vi "Time.vi"(8 "error in (no error)":errorcluster, 10 "Control In":T1, 11 "CAD Dispense in":refnum<class "CAD Dispense.lvclass">) -> (0 "error out":errorcluster, 1 "Timing Data":i32[](array[numeric]), 2 "Control Out":T1, 3 "CAD Dispense out":refnum<class "CAD Dispense.lvclass">)   [LabVIEW 2020, in "CAD Dispense.lvclass"]
uses:
  CAD Dispense.lvclass
  Controller/Motion/Motion.lvclass
  Controller/Controllers.ctl
  Controller/Controller.lvclass
  Controller/I-O/I-O.lvclass
  Controller/Dispenser/Dispenser.lvclass
  C:/Program Files (x86)/Aerotech/A3200/LabVIEW/2010/Bin/Aerotech.A3200.dll
  Program Files (x86)/Aerotech/A3200/LabVIEW/2010/Bin/Aerotech.A3200.dll
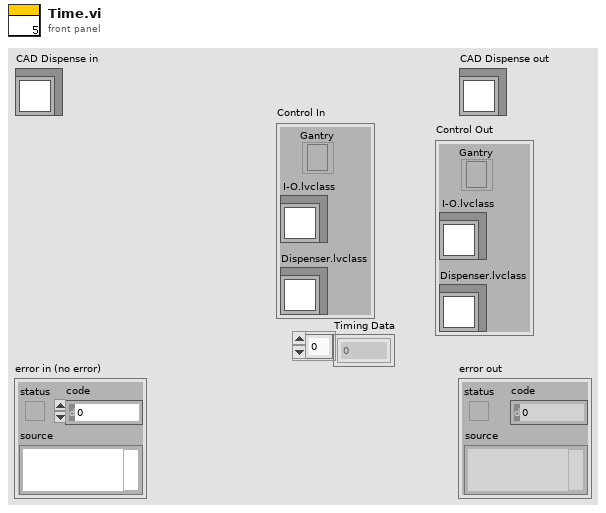
[diagram p1: front panel]
types:
  T1 = typedef "Controller.lvclass/Controllers.ctl" = cluster{"I-O.lvclass":refnum<class "I-O.lvclass">, "Dispenser.lvclass":refnum<class "Dispenser.lvclass">, "Gantry":refnum<k24>}
  T2 = cluster{"Motion":dbl[][], "Center":dbl[], "CW/CCW":dbl, "Dispense Type":enum16{"N-gon", "Square", "Arc", "Dot", "Line", "Circle"}}[]
  T3 = enum16{"N-gon", "Square", "Arc", "Dot", "Line", "Circle"}
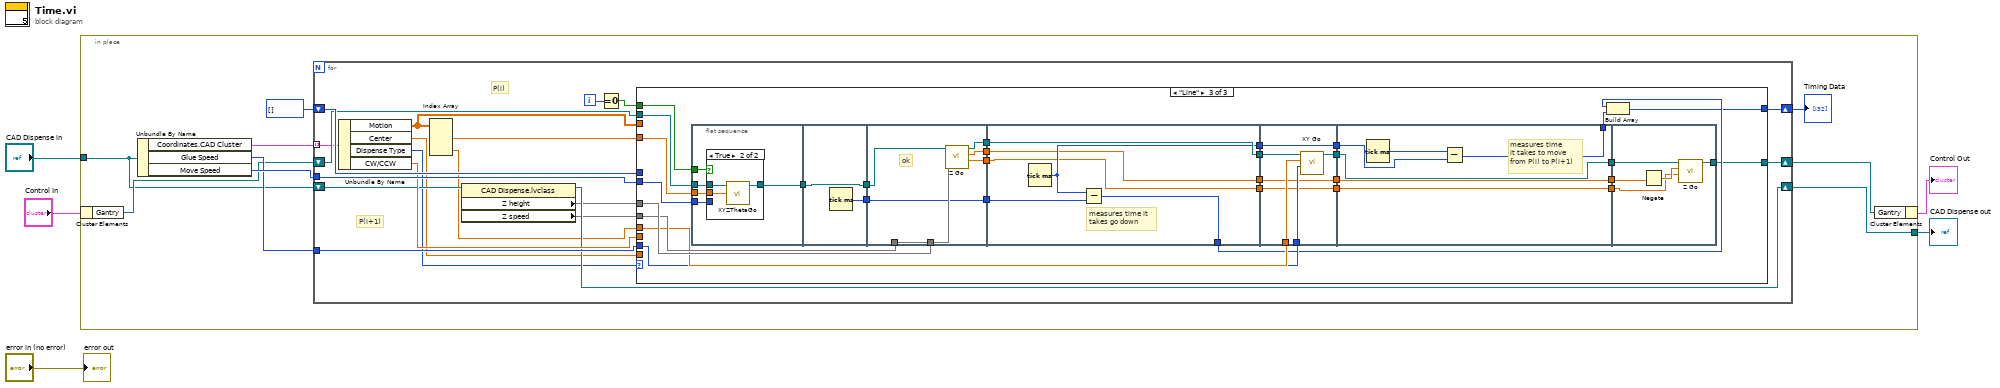
[diagram p0: block diagram]
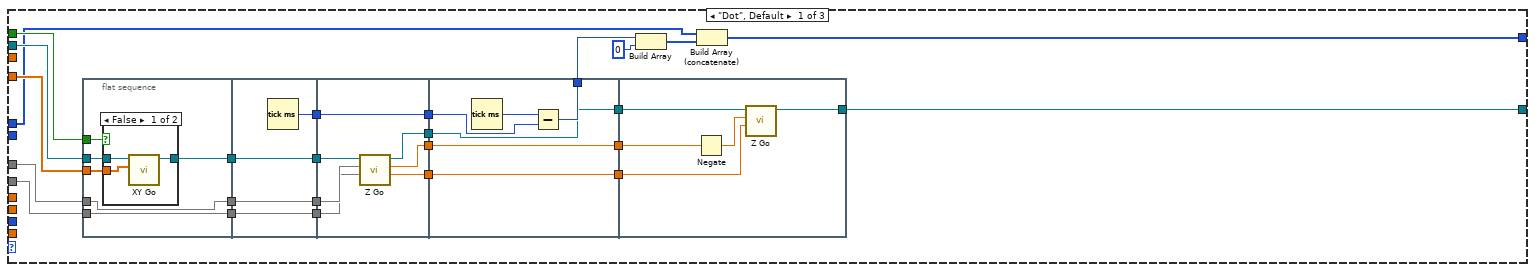
[diagram p2: hidden frame]
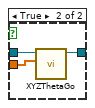
[diagram p3: hidden frame]
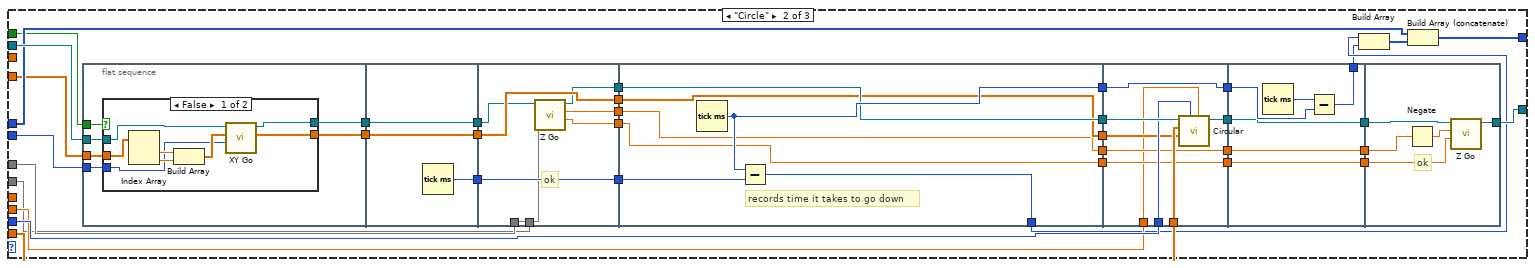
[diagram p4: hidden frame]
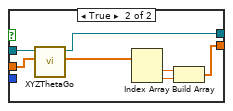
[diagram p5: hidden frame]
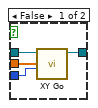
[diagram p6: hidden frame]
diagram:
  n1 = in-place {
    in-place-border: "CAD Dispense in" -> [w10]
    in-place-border: [w9] -> w1
    n2 = in-place-cluster #1("Control In") -> ("Gantry"=w11:refnum<k24>)
    n3 = Unbundle By Name "Unbundle By Name"(w10) -> ("Coordinates.CAD Cluster"=w6:T2, "Glue Speed"=w13:i32, "Move Speed"=w14:i32)
    n4 = for {
      tunnel: w14 -> [w33]
      shift-right: [w17] -> w7
      shift-left: w11 -> [w30]
      tunnel: w13 -> [w32]
      shift-right: [w22] -> w8
      shift-left: i32[] [] -> [w31]
      shift-right: [w27] -> w9
      shift-left: w10 -> [w28]
      tunnel: w6 -> [w21] mode=indexing
      i -> [w26]
      # "P(i+1)"
      # "P(i)"
      n5 = Unbundle By Name(w21) -> ("Motion"=w16:dbl[][], "Center"=w15:dbl[], "Dispense Type"=w20:T3, "CW/CCW"=w29:dbl)
      n6 = Index Array(array=w16) -> (element #1=w18:dbl[], element #2=w19:dbl[])  [unwired: 4 in]
      n7 = property class="CAD Dispense.lvclass"(reference=w28) -> (reference out=w27:refnum<class "CAD Dispense.lvclass">, "Z height"=w24, "Z speed"=w23)  [unwired: 1 in, 1 out]
      n8 = Equal To 0?(x=w26) -> (x = 0?=w25:bool)
      n9 = case shown="\"Line\"" w20 {
        tunnel: w15 -> [_ w117 _]
        tunnel: w30 -> [w52 w118 w218]
        tunnel: w33 -> [_ w106 w216]
        tunnel: [w34 w125 w189] -> w17
        tunnel: w32 -> [_ w116 w205]
        tunnel: w29 -> [_ w115 _]
        tunnel: w31 -> [w42 w112 _]
        tunnel: [w41 w110 w190] -> w22
        tunnel: w18 -> [w53 w105 w217]
        tunnel: w23 -> [w46 w108 w211]
        tunnel: w24 -> [w49 w109 w212]
        tunnel: w25 -> [w54 w107 w215]
        tunnel: w19 -> [_ _ w206]
        tunnel: w16 -> [_ _ _]
        frame "Dot", Default {
          n10 = flat-sequence {
            tunnel: w54 -> [w64]
            tunnel: w53 -> [w63]
            tunnel: w52 -> [w62]
            tunnel: [w61] -> w50
            tunnel: w49 -> [w60]
            tunnel: [w60] -> w47
            tunnel: w46 -> [w59]
            tunnel: [w59] -> w44
            tunnel: [w74] -> w58
            tunnel: [w73] -> w51
            tunnel: w50 -> [w73]
            tunnel: [w72] -> w48
            tunnel: w47 -> [w72]
            tunnel: [w71] -> w45
            tunnel: w44 -> [w71]
            tunnel: [w81] -> w57
            tunnel: w58 -> [w81]
            tunnel: w51 -> [w80]
            tunnel: w48 -> [w79]
            tunnel: w45 -> [w78]
            tunnel: [w77] -> w39
            tunnel: [w76] -> w37
            tunnel: [w75] -> w35
            tunnel: w57 -> [w87]
            tunnel: [w85] -> w56
            tunnel: [w84] -> w40
            tunnel: w39 -> [w84]
            tunnel: [w83] -> w38
            tunnel: w37 -> [w83]
            tunnel: [w82] -> w36
            tunnel: w35 -> [w82]
            tunnel: w40 -> [w92]
            tunnel: w38 -> [w90]
            tunnel: w36 -> [w89]
            tunnel: [w88] -> w34
            frame #0 {
              n11 = case shown="False" w64 {
                tunnel: w63 -> [w65 w70]
                tunnel: w62 -> [w67 w69]
                tunnel: [w66 w68] -> w61
                frame False {
                  n12 = call "XY Go.vi"("XY In"=w65, "Gantry"=w67) -> ("Gantry  2"=w66:refnum<k24>)  [unwired: 7 in, 2 out]
                }
                frame True {
                  n13 = call "XYZThetaGo.vi"("XYZTheta In"=w70, "Gantry"=w69) -> ("Gantry 3"=w68:refnum<k24>)  [unwired: 7 in, 2 out]
                }
              }
            }
            frame #1 {
              n14 = Tick Count (ms)() -> (millisecond timer value=w74:u32)
            }
            frame #2 {
              n15 = call "Z Go.vi"("Speed In"=w78, "Position In"=w79, "Gantry"=w80) -> ("Speed Out"=w76:dbl, "Position Out"=w77:dbl, "Gantry  2"=w75:refnum<k24>)  [unwired: 5 in, 1 out]
            }
            frame #3 {
              n16 = Tick Count (ms)() -> (millisecond timer value=w86:u32)
              n17 = Subtract(x=w86, y=w87) -> (x-y=w85:u32)
            }
            frame #4 {
              n18 = Negate(x=w92) -> (-x=w91:dbl)
              n19 = call "Z Go.vi"("Speed In"=w90, "Position In"=w91, "Gantry"=w89) -> ("Gantry  2"=w88:refnum<k24>)  [unwired: 5 in, 3 out]
            }
          }
          n20 = Build Array(w56, 0) -> (w55:u32[])
          n21 = Build Array (concatenate)(w42, w55) -> (w41:u32[])
        }
        frame "Circle" {
          n22 = flat-sequence {
            tunnel: [w132] -> w123
            tunnel: w118 -> [w133]
            tunnel: w105 -> [w134]
            tunnel: w107 -> [w135]
            tunnel: w106 -> [w131]
            tunnel: [w130] -> w101
            tunnel: [w153] -> w129
            tunnel: [w152] -> w124
            tunnel: w123 -> [w152]
            tunnel: [w151] -> w102
            tunnel: w101 -> [w151]
            tunnel: w129 -> [w161]
            tunnel: [w161] -> w128
            tunnel: w124 -> [w159]
            tunnel: [w158] -> w122
            tunnel: w109 -> [w157]
            tunnel: w108 -> [w156]
            tunnel: [w160] -> w103
            tunnel: w102 -> [w160]
            tunnel: [w155] -> w98
            tunnel: [w154] -> w95
            tunnel: w128 -> [w168]
            tunnel: [w167] -> w126
            tunnel: [w166] -> w114
            tunnel: w122 -> [w165]
            tunnel: [w165] -> w121
            tunnel: [w164] -> w104
            tunnel: w103 -> [w164]
            tunnel: [w163] -> w99
            tunnel: w98 -> [w163]
            tunnel: [w162] -> w96
            tunnel: w95 -> [w162]
            tunnel: [w177] -> w127
            tunnel: w126 -> [w177]
            tunnel: w121 -> [w176]
            tunnel: [w175] -> w119
            tunnel: w117 -> [w173]
            tunnel: w116 -> [w174]
            tunnel: w115 -> [w169]
            tunnel: w104 -> [w172]
            tunnel: [w171] -> w100
            tunnel: w99 -> [w171]
            tunnel: [w170] -> w97
            tunnel: w96 -> [w170]
            tunnel: w127 -> [w182]
            tunnel: [w181] -> w113
            tunnel: [w180] -> w120
            tunnel: w119 -> [w180]
            tunnel: w100 -> [w179]
            tunnel: w97 -> [w178]
            tunnel: [w179] -> w94
            tunnel: [w178] -> w93
            tunnel: [w186] -> w125
            tunnel: w120 -> [w187]
            tunnel: w94 -> [w188]
            tunnel: w93 -> [w185]
            frame #0 {
              n23 = case shown="False" w135 {
                tunnel: w134 -> [w143 w148]
                tunnel: w133 -> [w142 w150]
                tunnel: [w141 w149] -> w132
                tunnel: w131 -> [w137 _]
                tunnel: [w136 w144] -> w130
                frame False {
                  n24 = Index Array(array=w143) -> (element #1=w140:dbl, element #2=w139:dbl)  [unwired: 2 in]
                  n25 = Build Array(w140, w139) -> (w138:dbl[])
                  n26 = call "XY Go.vi"("Speed"=w137, "XY In"=w138, "Gantry"=w142) -> ("XY Out 2"=w136:dbl[], "Gantry  2"=w141:refnum<k24>)  [unwired: 6 in, 1 out]
                }
                frame True {
                  n27 = call "XYZThetaGo.vi"("XYZTheta In"=w148, "Gantry"=w150) -> ("XYZTheta Out"=w147:dbl[], "Gantry 3"=w149:refnum<k24>)  [unwired: 7 in, 1 out]
                  n28 = Index Array(array=w147) -> (element #1=w146:dbl, element #2=w145:dbl)  [unwired: 2 in]
                  n29 = Build Array(w146, w145) -> (w144:dbl[])
                }
              }
            }
            frame #1 {
              n30 = Tick Count (ms)() -> (millisecond timer value=w153:u32)
            }
            frame #2 {
              # "ok"
              n31 = call "Z Go.vi"("Speed In"=w156, "Position In"=w157, "Gantry"=w159) -> ("Speed Out"=w154:dbl, "Position Out"=w155:dbl, "Gantry  2"=w158:refnum<k24>)  [unwired: 5 in, 1 out]
            }
            frame #3 {
              # "records time it takes to go down"
              n32 = Tick Count (ms)() -> (millisecond timer value=w167:u32)
              n33 = Subtract(x=w167, y=w168) -> (x-y=w166:u32)
            }
            frame #4 {
              n34 = call "Circular.vi"("Direction"=w169, "Speed"=w174, "XY End"=w172, "XY Center"=w173, "Gantry"=w176) -> ("Gantry  2"=w175:refnum<k24>)  [unwired: 5 in, 1 out]
            }
            frame #5 {
              n35 = Tick Count (ms)() -> (millisecond timer value=w183:u32)
              n36 = Subtract(x=w183, y=w182) -> (x-y=w181:u32)
            }
            frame #6 {
              # "ok"
              n37 = Negate(x=w188) -> (-x=w184:dbl)
              n38 = call "Z Go.vi"("Speed In"=w185, "Position In"=w184, "Gantry"=w187) -> ("Gantry  2"=w186:refnum<k24>)  [unwired: 5 in, 3 out]
            }
          }
          n39 = Build Array(w114, w113) -> (w111:u32[])
          n40 = Build Array (concatenate)(w112, w111) -> (w110:u32[])
        }
        frame "Line" {
          n41 = flat-sequence {
            tunnel: w218 -> [w223]
            tunnel: w217 -> [w222]
            tunnel: w216 -> [w221]
            tunnel: w215 -> [w220]
            tunnel: [w219] -> w214
            tunnel: w214 -> [w232]
            tunnel: [w232] -> w213
            tunnel: [w231] -> w209
            tunnel: w213 -> [w239]
            tunnel: w212 -> [w238]
            tunnel: w211 -> [w237]
            tunnel: [w236] -> w210
            tunnel: w209 -> [w236]
            tunnel: [w235] -> w207
            tunnel: [w234] -> w197
            tunnel: [w233] -> w193
            tunnel: w210 -> [w245]
            tunnel: [w244] -> w192
            tunnel: [w243] -> w208
            tunnel: w207 -> [w243]
            tunnel: [w242] -> w203
            tunnel: [w241] -> w198
            tunnel: w197 -> [w241]
            tunnel: [w240] -> w194
            tunnel: w193 -> [w240]
            tunnel: w208 -> [w252]
            tunnel: w206 -> [w251]
            tunnel: w205 -> [w250]
            tunnel: [w249] -> w204
            tunnel: w203 -> [w249]
            tunnel: [w248] -> w201
            tunnel: [w247] -> w199
            tunnel: w198 -> [w247]
            tunnel: [w246] -> w195
            tunnel: w194 -> [w246]
            tunnel: w204 -> [w257]
            tunnel: [w256] -> w191
            tunnel: [w255] -> w202
            tunnel: w201 -> [w255]
            tunnel: [w254] -> w200
            tunnel: w199 -> [w254]
            tunnel: [w253] -> w196
            tunnel: w195 -> [w253]
            tunnel: w202 -> [w263]
            tunnel: w200 -> [w262]
            tunnel: w196 -> [w260]
            tunnel: [w259] -> w189
            frame #0 {
              n42 = case shown="True" w220 {
                tunnel: w223 -> [w227 w229]
                tunnel: w222 -> [w226 w230]
                tunnel: w221 -> [w225 _]
                tunnel: [w224 w228] -> w219
                frame False {
                  n43 = call "XY Go.vi"("Speed"=w225, "XY In"=w226, "Gantry"=w227) -> ("Gantry  2"=w224:refnum<k24>)  [unwired: 6 in, 2 out]
                }
                frame True {
                  n44 = call "XYZThetaGo.vi"("XYZTheta In"=w230, "Gantry"=w229) -> ("Gantry 3"=w228:refnum<k24>)  [unwired: 7 in, 2 out]
                }
              }
            }
            frame #1 {
              n45 = Tick Count (ms)() -> (millisecond timer value=w231:u32)
            }
            frame #2 {
              # "ok"
              n46 = call "Z Go.vi"("Speed In"=w237, "Position In"=w238, "Gantry"=w239) -> ("Speed Out"=w233:dbl, "Position Out"=w234:dbl, "Gantry  2"=w235:refnum<k24>)  [unwired: 5 in, 1 out]
            }
            frame #3 {
              # "measures time it \ntakes go down"
              n47 = Tick Count (ms)() -> (millisecond timer value=w242:u32)
              n48 = Subtract(x=w242, y=w245) -> (x-y=w244:u32)
            }
            frame #4 {
              n49 = call "XY Go.vi"("Speed"=w250, "XY In"=w251, "Gantry"=w252) -> ("Gantry  2"=w248:refnum<k24>)  [unwired: 6 in, 2 out]
            }
            frame #5 {
              # "measures time\nit takes to move\nfrom P(i) to P(i+1)"
              n50 = Tick Count (ms)() -> (millisecond timer value=w258:u32)
              n51 = Subtract(x=w258, y=w257) -> (x-y=w256:u32)
            }
            frame #6 {
              n52 = Negate(x=w262) -> (-x=w261:dbl)
              n53 = call "Z Go.vi"("Speed In"=w260, "Position In"=w261, "Gantry"=w263) -> ("Gantry  2"=w259:refnum<k24>)  [unwired: 5 in, 3 out]
            }
          }
          n54 = Build Array(w192, w191) -> (w190:u32[])
        }
      }
    }
    "Timing Data" <- w8
    n55 = in-place-cluster #1("Gantry"=w7) -> (→"Control Out":T1)
  }
  "CAD Dispense out" <- w1
  "error out" <- "error in (no error)"
